vi "Wavelet Packet - Read and Write Coefficients.vi"() -> ()   [LabVIEW 2023]
doc: "This example shows how to read and write the coefficients of a certain node of a wavelet packet tree with the WA WP Read Node VI and the WA WP Write Node VI, respectively.\n\n<b>Instructions:</b>\n1) Run this VI.\n2) Observe the <b>Node Coefficients</b>.\n3) Change the value of <b>Path</b> to obtain the coefficients at other nodes.\n4) Browse the Block Diagram to learn how to read and write coefficients from and to a wavelet packet tree."
uses:
  <vilib>/addons/Wavelet Analysis/wavelet packet.llb/WA WP Decomposition (Waveform).vi
  <vilib>/addons/Wavelet Analysis/wavelet packet.llb/WA WP Reconstruction (Waveform).vi
  <vilib>/addons/_Advanced Signal Processing/NI_AdvSigProcWA.lvlib
panel:
  in  "Data":u16(ring)=115 items=["1D Example Data"=100, "-"=101, "Doppler"=102, "HOP"=103, "TF Sine"=104, "Noisy Doppler"=105, "Sea Temperature"=106, "Sp500"=107, "Power Line"=108, "Engine Knocking"=109, "HeaviSine"=110, "Bumps"=111, "Blocks"=112, "Piece Regular"=113, "HypChirps"=114, "LinChirps"=115, "Chirps"=116, "Piece Polynomial"=117, "ECG"=131, "-"=118, "2D Example Data"=119, "-"=120, "Finger Print (Image)"=121, "Iris Flower (Image)"=122, "Mammogram (Image)"=123, "Lake (Image)"=127, "Two Can 1 (Image)"=132, "Two Can 2 (Image)"=133, "Camera Man (Image)"=134]
  out "aspt-left-top":bool
  in  "Levels":i32=4
  in  "stop":bool
  out "Node Coefficients":dbl[](graph)
  out "Reconstructed Signal":waveform(dbl)(graph)
  out "Signal":waveform(dbl)(graph)
  in  "Path":string="0001"
  in  "Wavelet":u16(ring) items=["db02"=0, "db03"=1, "db04"=2, "db05"=3, "db06"=4, "db07"=5, "db08"=6, "db09"=7, "db10"=8, "db11"=9, "db12"=10, "db13"=11, "db14"=12, "Haar"=13, "bior1_3"=14, "bior1_5"=15, "bior2_2"=16, "bior2_4"=17, "bior2_6"=18, "bior2_8"=19, "bior3_1"=20, "bior3_3"=21, "bior3_5"=22, "bior3_7"=23, "bior3_9"=24, "bior4_4 (FBI)"=25, "bior5_5"=38, "bior6_8"=39, "coif1"=26, "coif2"=27, "coif3"=28, "coif4"=29, "coif5"=30, "sym2"=31, "sym3"=32, "sym4"=33, "sym5"=34, "sym6"=35, "sym7"=36, "sym8"=37]
  # "Overview: Shows how to read and write the coefficients of a certain node of a wavelet packet tree with the WA WP Read Node VI and the WA WP Write Node VI, respectively.\nRequirements: LabVIEW Full Development System, Advanced Signal Processing Toolkit\nInstructions: \n1. Run this VI.\n2. Observe the Node Coefficients.\n3. Change the value of Path to obtain the coefficients at other nodes.\n4. Browse the Block Diagram to learn how to read and write coefficients from and to a wavelet packet tree.\n5. Click Stop to stop the VI."
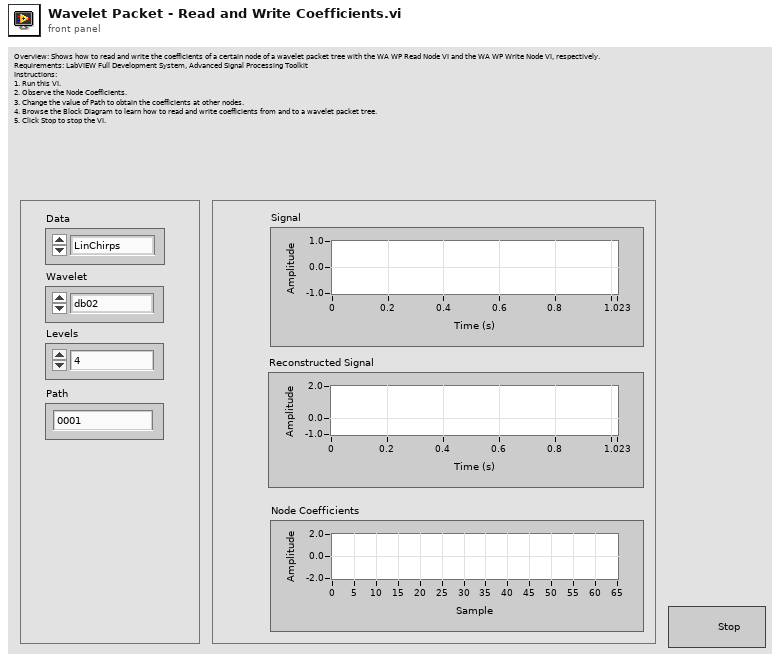
[diagram p1: front panel]
types:
  T1 = typedef "NI_AdvSigProcWA.lvlib/WA Generic Ref.ctl" = cluster{"ref":u64, "t0":timestamp, "dt":dbl}
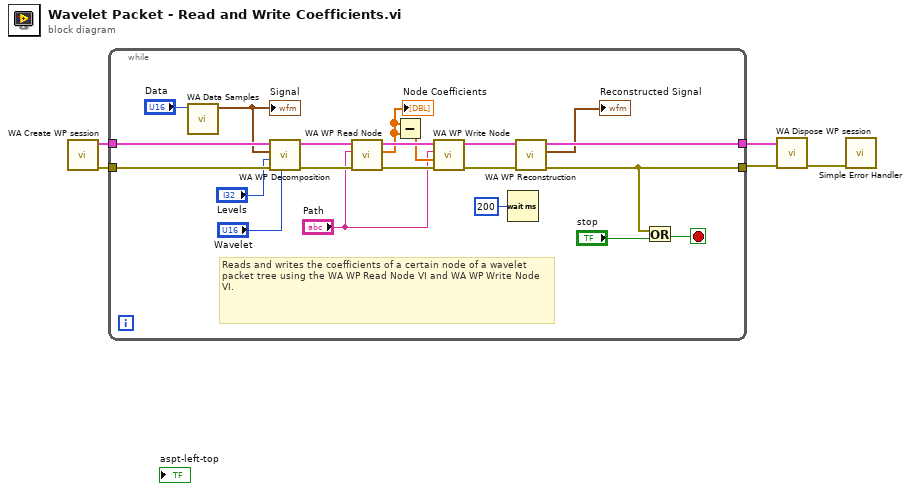
[diagram p0: block diagram]
diagram:
  n1 = call <vilib>:"WA Create WP session.vi"() -> ("error out"=w4:errorcluster, "WP session out"=w5:T1)  [unwired: 1 in, 9 out]
  n2 = while {
    tunnel: w5 -> [w26]
    tunnel: w4 -> [w25]
    tunnel: [w18] -> w3
    tunnel: [w6] -> w2
    stop <- w9 stop-if-true
    # "Reads and writes the coefficients of a certain node of a wavelet packet tree using the WA WP Read Node VI and WA WP Write Node VI."
    n3 = call <vilib>:"WA Data Samples.vi"("data"="Data") -> ("signal"=w15:waveform(dbl))  [unwired: 10 out]
    "Signal" <- w15
    n4 = call-poly <vilib>:"WA WP Decomposition.vi"("wavelet"="Wavelet", "error in (no error)"=w25, "levels"="Levels", "signal"=w15, "WP session"=w26) -> ("error out"=w23:errorcluster, "WP session out"=w24:T1)  [unwired: 5 out]
    n5 = call <vilib>:"WA WP Read Node.vi"("error in (no error)"=w23, "path"="Path", "WP session"=w24) -> ("error out"=w22:errorcluster, "node coef"=w13:dbl[], "WP session out"=w21:T1)  [unwired: 1 in, 5 out]
    "Node Coefficients" <- w13
    n6 = Subtract(x=w13, y=w13) -> (x-y=w12:dbl[])
    n7 = call <vilib>:"WA WP Write Node.vi"("error in (no error)"=w22, "node coef"=w12, "path"="Path", "WP session"=w21) -> ("error out"=w19:errorcluster, "WP session out"=w20:T1)  [unwired: 6 out]
    n8 = Wait (ms)(milliseconds to wait=u32 200 ("millisecond multiple")) -> ()  [unwired: 1 out]
    n9 = call-poly <vilib>:"WA WP Reconstruction.vi"("error in (no error)"=w19, "WP session"=w20) -> ("error out"=w6:errorcluster, "signal"=→"Reconstructed Signal":waveform(dbl), "WP session out"=w18:T1)  [unwired: 7 out]
    n10 = Or(x=w6, y="stop") -> (x .or. y?=w9:bool)
  }
  n11 = call <vilib>:"WA Dispose WP session.vi"("error in (no error)"=w2, "WP session"=w3) -> ("error out"=w1:errorcluster)  [unwired: 9 out]
  n12 = call <vilib>:"Simple Error Handler.vi"("error in (no error)"=w1) -> ()  [unwired: 1 in, 8 out]
